vi "girpcutil_RpcValue_GetSize.vi"(5 "param handle":i32, 7 "member":string, 8 "Fehler (Eingang, kein Fehler)":errorcluster, 11 "girpcutil_params":T1) -> (0 "Fehler (Ausgang)":errorcluster, 2 "size":u64)   [LabVIEW 2016]
uses:
  girpcutil_params.ctl
panel:
  out "errMsg 2":u8[](array[numeric])
  out "errMsgLen 2":i32
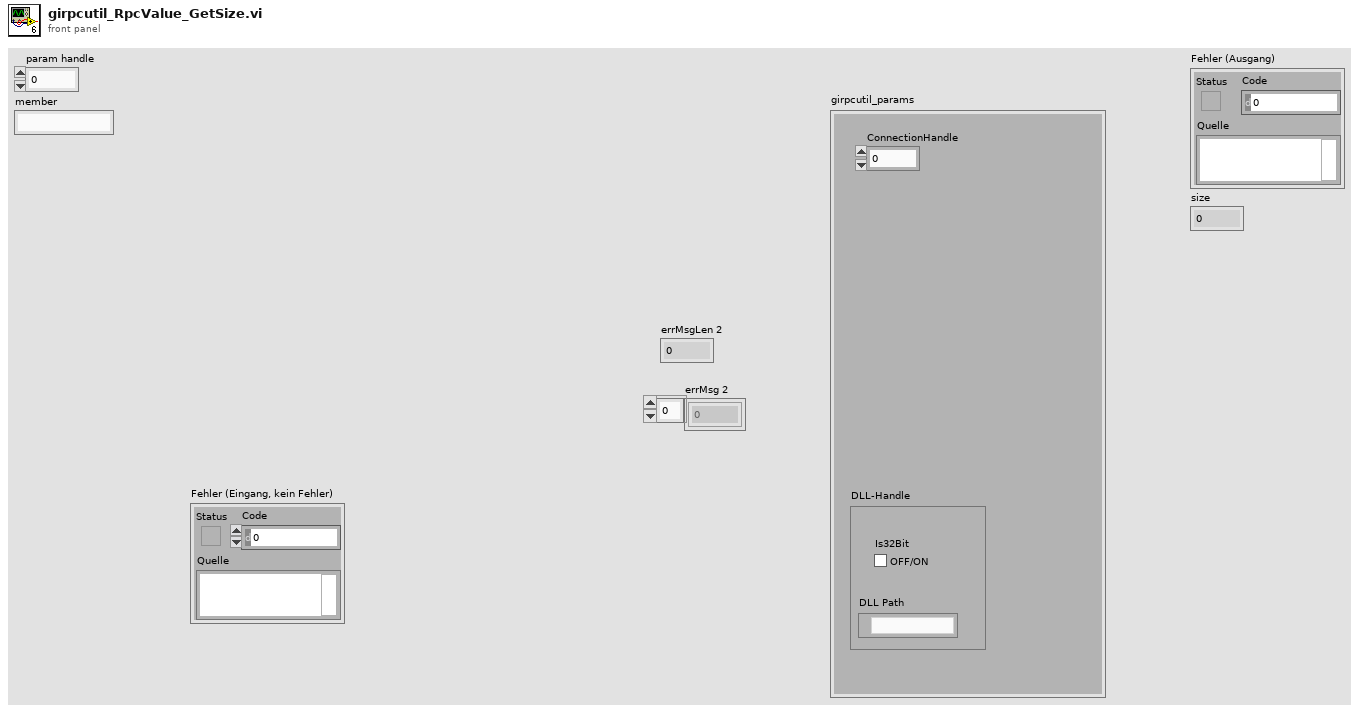
[diagram p1: front panel]
types:
  T1 = typedef "girpcutil_params.ctl" = cluster{"ConnectionHandle":i32, "DLL-Handle":cluster{"DLL Path":path, "Is32Bit":bool}}
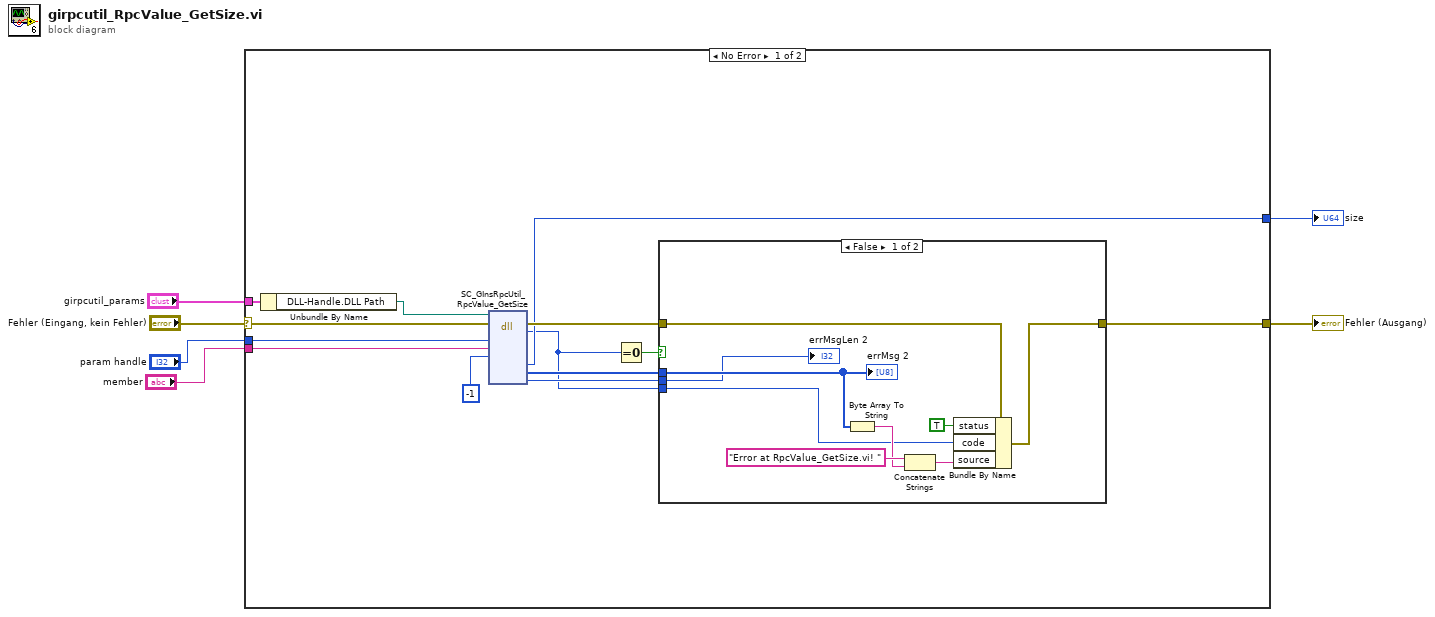
[diagram p0: block diagram]
diagram:
  n1 = case shown="No Error" "Fehler (Eingang, kein Fehler)" {
    selector: "Fehler (Eingang, kein Fehler)" -> [w19 w30]
    tunnel: [w12 w30] -> w5
    tunnel: "girpcutil_params" -> [w18 _]
    tunnel: "param handle" -> [w16 _]
    tunnel: "member" -> [w15 _]
    tunnel: [w11 _] -> w1
    frame No Error {
      n2 = Unbundle By Name(w18) -> ("DLL-Handle.DLL Path"=w17:path)
      n3 = dll-call lib="?" fn="SC_GInsRpcUtil_RpcValue_GetSize"(path in=w17, error in=w19, "value"=w16, "member"=w15, "index"=-1) -> (error out=w13:errorcluster, "Rückgabewert"=w7:i32, "size"=w11:u64, "errMsg"=w9:u8[], "errMsgLen"=w10:i32)  [unwired: 7 in, 1 out]
      n4 = Equal To 0?(x=w7) -> (x = 0?=w8:bool)
      n5 = case shown="False" w8 {
        tunnel: w13 -> [w22 w29]
        tunnel: [w21 w29] -> w12
        tunnel: w9 -> [w26 _]
        tunnel: w10 -> [w23 _]
        tunnel: w7 -> [w20 _]
        frame False {
          n6 = Byte Array To String(unsigned byte array=w26) -> (string=w27:string)
          n7 = Concatenate Strings("Error at RpcValue_GetSize.vi! " ("source"), w27) -> (w25:string)
          n8 = Bundle By Name(cluster=w22, "status"=TRUE, "code"=w20, "source"=w25) -> (w21:errorcluster)
          "errMsg 2" <- w26
          "errMsgLen 2" <- w23
        }
        frame True {
        }
      }
    }
    frame Error {
    }
  }
  "Fehler (Ausgang)" <- w5
  "size" <- w1
